vi "Read Application.vi"(8 "error in (no error)":errorcluster, 11 "Application Interface in":refnum<class "Application Interface.lvclass">) -> (0 "error out":errorcluster, 2 "Application.lvclass":refnum<class "Application.lvclass">, 3 "Application Interface out":refnum<class "Application Interface.lvclass">)   [LabVIEW 2016, in "Application Interface.lvclass"]
uses:
  Application Interface.lvclass
  Application.lvclass
  Application Interface.lvclass/Application Interface.ctl
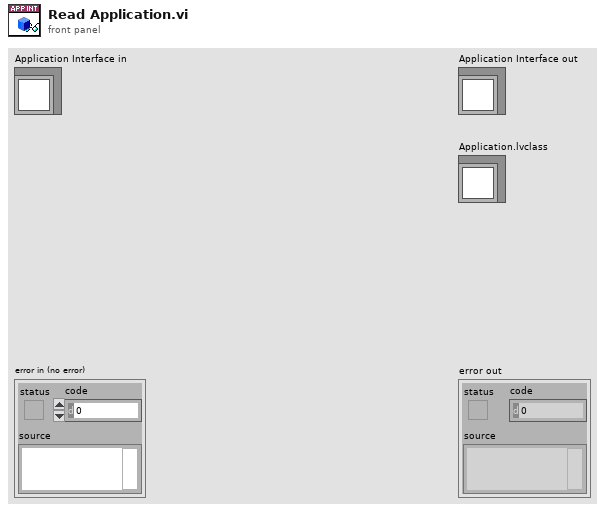
[diagram p1: front panel]
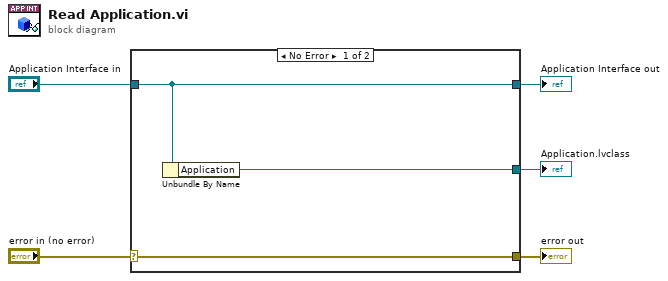
[diagram p0: block diagram]
diagram:
  n1 = case shown="No Error" "error in (no error)" {
    selector: "error in (no error)" -> [w8 w9]
    tunnel: [w8 w9] -> w4
    tunnel: [w7 w10] -> w2
    tunnel: "Application Interface in" -> [w7 w10]
    tunnel: [w6 _] -> w1
    frame No Error {
      n2 = Unbundle By Name(w7) -> ("Application"=w6:refnum<class "Application.lvclass">)
    }
    frame Error {
    }
  }
  "error out" <- w4
  "Application Interface out" <- w2
  "Application.lvclass" <- w1
